vi "output_waveforms_from_DAQ.vi"(5 "Laser":u16, 8 "DO data":digitalwaveform[](array[waveform]), 9 "AO data":waveform(dbl)[](array[waveform]), 10 "rate":dbl=1000.0 format="%0.2f", 11 "samples per channel":i32=1000) -> ()   [LabVIEW 2013]
uses:
  <vilib>/DAQmx/configure/timing.llb/DAQmx Timing (Sample Clock).vi
  <vilib>/DAQmx/create/channels.llb/DAQmx Create Channel (DO-Digital Output).vi
  <vilib>/DAQmx/create/channels.llb/DAQmx Create Channel (AO-Voltage-Basic).vi
  <vilib>/DAQmx/configure/trigger.llb/DAQmx Start Trigger (Digital Edge).vi
  <vilib>/DAQmx/write.llb/DAQmx Write (Analog 1D Wfm NChan NSamp).vi
  <vilib>/DAQmx/write.llb/DAQmx Write (Digital 1D Wfm NChan NSamp).vi
  <vilib>/DAQmx/create/channels.llb/DAQmx Create Channel (CO-Pulse Generation-Time).vi
  <vilib>/Utility/error.llb/DialogType.ctl
  <vilib>/DAQmx/write.llb/DAQmx Write (Digital Bool 1Line 1Point).vi
panel:
  in  "minimum value":dbl=-10.0 caption="Output Minimum Value" format="%0.2f"
  in  "maximum value":dbl=10.0 caption="Output Maximum Value" format="%0.2f"
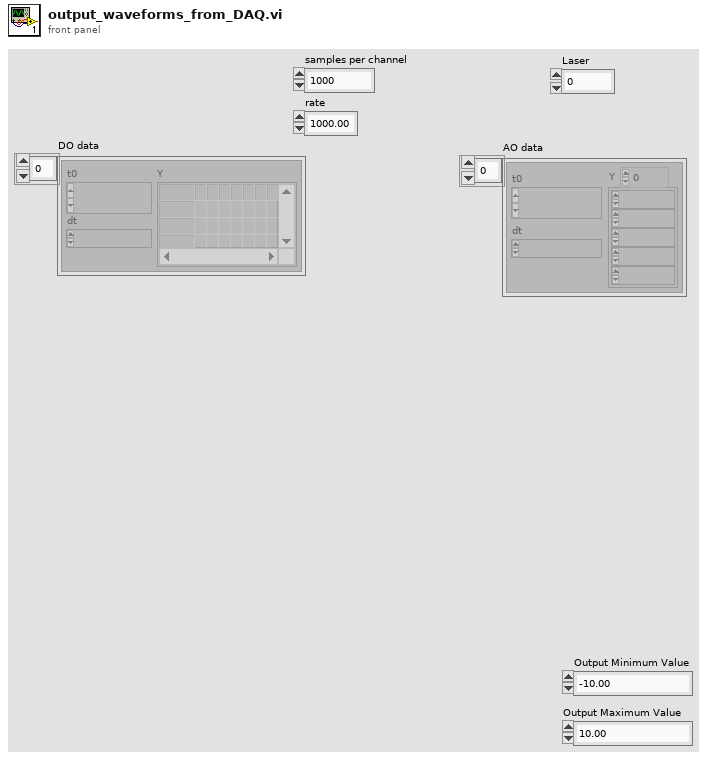
[diagram p1: front panel]
types:
  T1 = typedef "DialogType.ctl" = u16
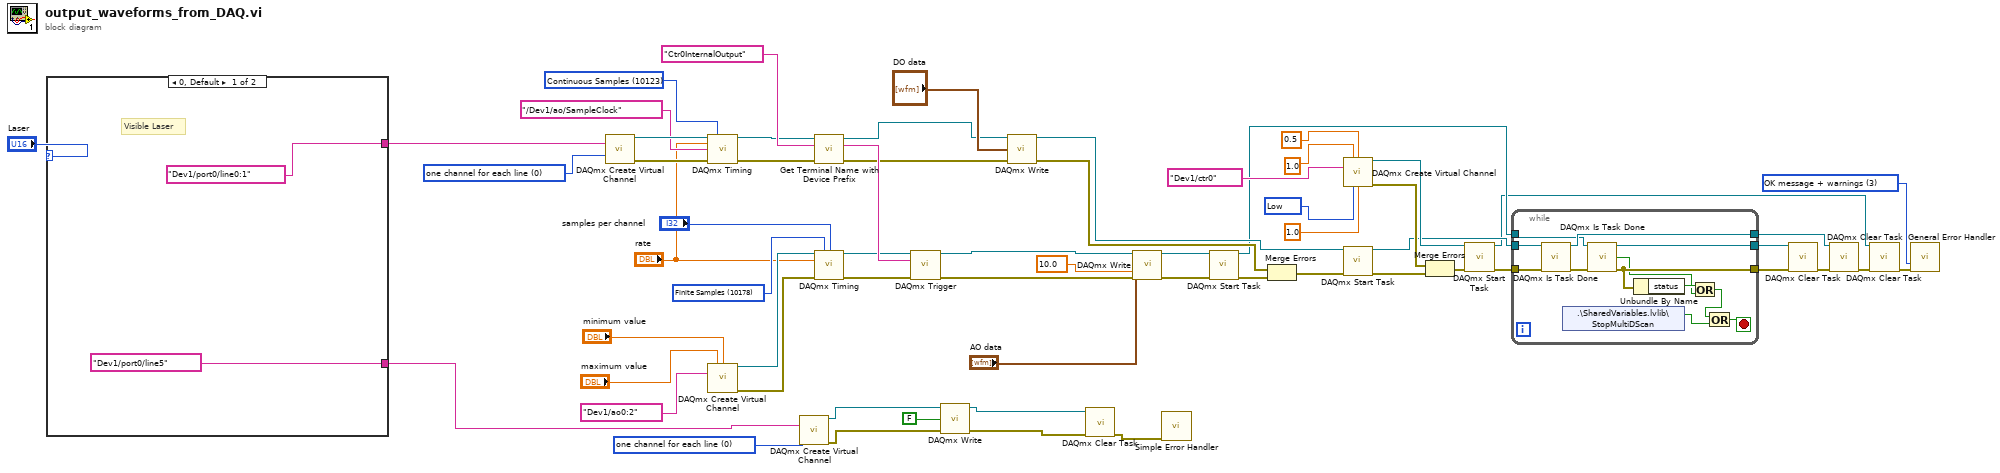
[diagram p0: block diagram]
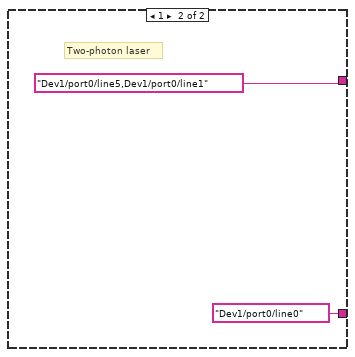
[diagram p2: hidden frame]
diagram:
  w8 = 0 items=["one channel for each line", "one channel for all lines"] ("line grouping")
  w17 = 0 items=["one channel for each line", "one channel for all lines"] ("line grouping")
  w26 = T1 3 items=["no dialog", "OK message", "continue or stop message", "OK message + warnings", "continue/stop + warnings"] ("type of dialog (OK msg:1)")
  w37 = 10214 items=["High"=10192, "Low"=10214] ("Idle State")
  w54 = 10178 items=["Finite Samples"=10178, "Continuous Samples"=10123] ("sample mode")
  w59 = 10123 items=["Finite Samples"=10178, "Continuous Samples"=10123] ("sample mode")
  n1 = case shown="0, Default" "Laser" {
    tunnel: [tag "Dev1/port0/line0:1" ("Physical Channel") tag "Dev1/port0/line5,Dev1/port0/line1" ("lines")] -> w9
    tunnel: [tag "Dev1/port0/line5" ("lines") tag "Dev1/port0/line0" ("lines")] -> w7
    frame 0, Default {
      # "Visible Laser"
    }
    frame 1 {
      # "Two-photon laser"
    }
  }
  n2 = call-poly <vilib>:"DAQmx Create Virtual Channel.vi"("lines"=w9, "line grouping"=w17) -> ("task out"=w57:refnum<k21>, "error out"=w58:errorcluster)  [unwired: 5 in, 7 out]
  n3 = call-poly <vilib>:"DAQmx Timing.vi"("task/channels in"=w57, "sample mode"=w59, "rate"="rate", "source"=tag "/Dev1/ao/SampleClock", "error in"=w58) -> ("task out"=w14:refnum<k21>, "error out"=w13:errorcluster)  [unwired: 2 in, 7 out]
  n4 = call-poly <vilib>:"DAQmx Create Virtual Channel.vi"("maximum value"="maximum value", "minimum value"="minimum value", "physical channels"=tag "Dev1/ao0:2") -> ("task out"=w53:refnum<k21>, "error out"=w52:errorcluster)  [unwired: 6 in, 5 out]
  n5 = call-poly <vilib>:"DAQmx Create Virtual Channel.vi"("lines"=w7, "line grouping"=w8) -> ("task out"=w6:refnum<k21>, "error out"=w5:errorcluster)  [unwired: 12 in]
  n6 = call "Get Terminal Name with Device Prefix.vi"("error in (no error)"=w13, "Local Terminal Name"="Ctr0InternalOutput" ("terminal"), "task/channels in"=w14) -> ("error out"=w40:errorcluster, "Terminal Name with Device Prefix"=w45:tag, "task out"=w41:refnum<k21>)  [unwired: 1 in, 5 out]
  n7 = call-poly <vilib>:"DAQmx Timing.vi"("task/channels in"=w53, "sample mode"=w54, "samples per channel"="samples per channel", "rate"="rate", "error in"=w52) -> ("task out"=w16:refnum<k21>, "error out"=w15:errorcluster)  [unwired: 2 in, 7 out]
  n8 = call-poly <vilib>:"DAQmx Trigger.vi"("task/channels in"=w16, "source"=w45, "error in"=w15) -> ("task out"=w47:refnum<k21>, "error out"=w48:errorcluster)  [unwired: 2 in, 9 out]
  n9 = call-poly <vilib>:"DAQmx Write.vi"("task/channels in"=w6, "data"=FALSE, "error in"=w5) -> ("task out"=w4:refnum<k21>, "error out"=w3:errorcluster)  [unwired: 10 in, 1 out]
  n10 = call-poly <vilib>:"DAQmx Write.vi"("task/channels in"=w41, "data"="DO data", "error in"=w40) -> ("task out"=w38:refnum<k21>, "error out"=w39:errorcluster)  [unwired: 2 in, 9 out]
  n11 = call <vilib>:"DAQmx Clear Task.vi"("task in"=w4, "error in"=w3) -> ("error out"=w2:errorcluster)  [unwired: 13 in]
  n12 = call-poly <vilib>:"DAQmx Write.vi"("task/channels in"=w47, "data"="AO data", "timeout"=10.0 ("Wirite Timeout"), "error in"=w48) -> ("task out"=w50:refnum<k21>, "error out"=w49:errorcluster)  [unwired: 1 in, 9 out]
  n13 = call <vilib>:"Simple Error Handler.vi"("error in (no error)"=w2) -> ()  [unwired: 4 in, 5 out]
  n14 = call <vilib>:"DAQmx Start Task.vi"("task/channels in"=w50, "error in"=w49) -> ("task out"=w21:refnum<k21>, "error out"=w44:errorcluster)  [unwired: 12 out]
  n15 = Merge Errors(w39, w44) -> (w43:errorcluster)
  n16 = call-poly <vilib>:"DAQmx Create Virtual Channel.vi"("high time"=1.0 ("High Time"), "low time"=0.5 ("Low Time"), "counter"=tag "Dev1/ctr0" ("Counter(s)"), "idle state"=w37, "initial delay"=1.0 ("Initial Delay")) -> ("task out"=w32:refnum<k21>, "error out"=w30:errorcluster)  [unwired: 4 in, 5 out]
  n17 = call <vilib>:"DAQmx Start Task.vi"("task/channels in"=w38, "error in"=w43) -> ("task out"=w20:refnum<k21>, "error out"=w31:errorcluster)  [unwired: 12 out]
  n18 = Merge Errors(w30, w31) -> (w29:errorcluster)
  n19 = call <vilib>:"DAQmx Start Task.vi"("task/channels in"=w32, "error in"=w29) -> ("task out"=w18:refnum<k21>, "error out"=w19:errorcluster)  [unwired: 12 out]
  n20 = while {
    tunnel: [w78] -> w28
    tunnel: w21 -> [w75]
    tunnel: [w74] -> w27
    tunnel: w20 -> [w73]
    tunnel: w19 -> [w72]
    tunnel: [w71] -> w25
    stop <- w68 stop-if-true
    n21 = call <vilib>:"DAQmx Is Task Done.vi"("task/channels in"=w73, "error in"=w72) -> ("task out"=w78:refnum<k21>, "error out"=w76:errorcluster)  [unwired: 2 in, 10 out]
    n22 = shared-variable ".\\SharedVariables.lvlib\\StopMultiDScan"() -> (w67:bool)  [unwired: 1 in, 1 out]
    n23 = call <vilib>:"DAQmx Is Task Done.vi"("task/channels in"=w75, "error in"=w76) -> ("task out"=w74:refnum<k21>, "task done?"=w70:bool, "error out"=w71:errorcluster)  [unwired: 11 out]
    n24 = Unbundle By Name(w71) -> ("status"=w77:bool)
    n25 = Or(x=w77, y=w70) -> (x .or. y?=w69:bool)
    n26 = Or(x=w69, y=w67) -> (x .or. y?=w68:bool)
  }
  n27 = call <vilib>:"DAQmx Clear Task.vi"("task in"=w27, "error in"=w25) -> ("error out"=w24:errorcluster)  [unwired: 13 out]
  n28 = call <vilib>:"DAQmx Clear Task.vi"("task in"=w28, "error in"=w24) -> ("error out"=w23:errorcluster)  [unwired: 13 out]
  n29 = call <vilib>:"DAQmx Clear Task.vi"("task in"=w18, "error in"=w23) -> ("error out"=w22:errorcluster)  [unwired: 13 out]
  n30 = call <vilib>:"General Error Handler.vi"("type of dialog (OK msg:1)"=w26, "error in (no error)"=w22) -> ()  [unwired: 1 in, 13 out]
